vi "Initialize Library.vi"(8 "error in":errorcluster, 11 "Log Producer in":refnum<class "Log Producer.lvclass">) -> (0 "error out":errorcluster, 3 "Log Producer out":refnum<class "Log Producer.lvclass">)   [LabVIEW 2020, in "AIM ARINC 664 Engine.lvlib" / "Implementation.lvlib" / "Frame Logging.lvlib" / "Log Producer.lvclass"]
uses:
  Log Producer.lvclass
  Log Producer.lvclass/Log Producer.ctl
  Logger Interface/Logger Interface.lvclass
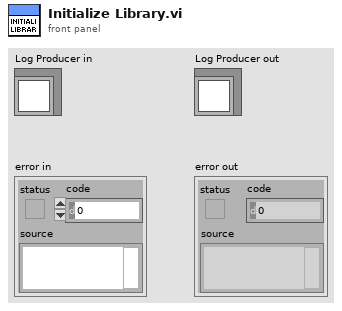
[diagram p1: front panel]
types:
  T1 = typedef "AIM ARINC 664 Engine.lvlib/Implementation.lvlib/Frame Logging.lvlib/Logger Data Reference.ctl" = refnum<data-value>
  T2 = cluster{"Logger Interface.lvclass":refnum<class "Logger Interface.lvclass">}
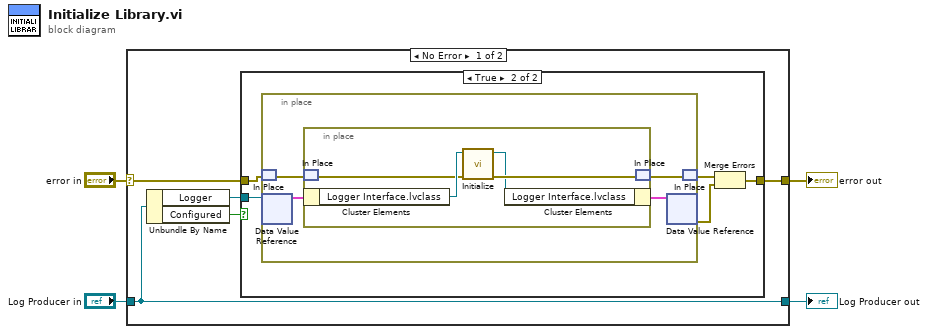
[diagram p0: block diagram]
diagram:
  n1 = case shown="No Error" "error in" {
    selector: "error in" -> [w9 w25]
    tunnel: [w7 w25] -> w3
    tunnel: [w5 w24] -> w1
    tunnel: "Log Producer in" -> [w5 w24]
    frame No Error {
      n2 = Unbundle By Name(w5) -> ("Logger"=w8:T1, "Configured"=w6:bool)
      n3 = case shown="True" w6 {
        tunnel: w9 -> [w10 w15]
        tunnel: w8 -> [_ w14]
        tunnel: [w10 w12] -> w7
        frame False {
        }
        frame True {
          n4 = in-place {
            n5 = in-place-match #1(w15) -> (w19:errorcluster)
            n6 = in-place-dvr #2(w14) -> (w17:T2)  [unwired: 1 out]
            n7 = in-place {
              n8 = in-place-match #3(w19) -> (w22:errorcluster)
              n9 = in-place-cluster #4(w17) -> ("Logger Interface.lvclass"=w23:refnum<class "Logger Interface.lvclass">)
              n10 = call-dynamic "Initialize.vi"("error in"=w22, "Logger Interface in"=w23) -> ("error out"=w21:errorcluster, "Logger Interface out"=w20:refnum<class "Logger Interface.lvclass">)  [unwired: 8 in]
              n11 = in-place-cluster #4("Logger Interface.lvclass"=w20) -> (w16:T2)
              n12 = in-place-match #3(w21) -> (w18:errorcluster)
            }
            n13 = in-place-dvr #2(w16) -> (w11:errorcluster)  [unwired: 1 out]
            n14 = in-place-match #1(w18) -> (w13:errorcluster)
          }
          n15 = Merge Errors(w13, w11) -> (w12:errorcluster)
        }
      }
    }
    frame Error {
    }
  }
  "error out" <- w3
  "Log Producer out" <- w1
